vi "Get settings chain.vi"(8 "error in (no error)":errorcluster, 11 "Cascade512Base in":refnum<class "DAQCascade512.lvclass">) -> (0 "error out":errorcluster, 1 "class name":string[](array[string]), 2 "settings":variant[](array[variant]), 3 "Cascade512Base out":refnum<class "DAQCascade512.lvclass">)   [LabVIEW 2012, in "DAQCascade512.lvclass"]
doc: "Returns an array of variants containing the settings clusters of each class in the inheritance chain (lowest child class first), together with an array of all class names in the inheritance chain.\n\nFor classes without settings cluster, the settings chain contains empty variants."
uses:
  DAQCascade512.lvclass
  <vilib>/Distrio/Murmex/Murmex/Murmex.lvclass
  DAQCascade512.lvclass/DAQCascade512.ctl
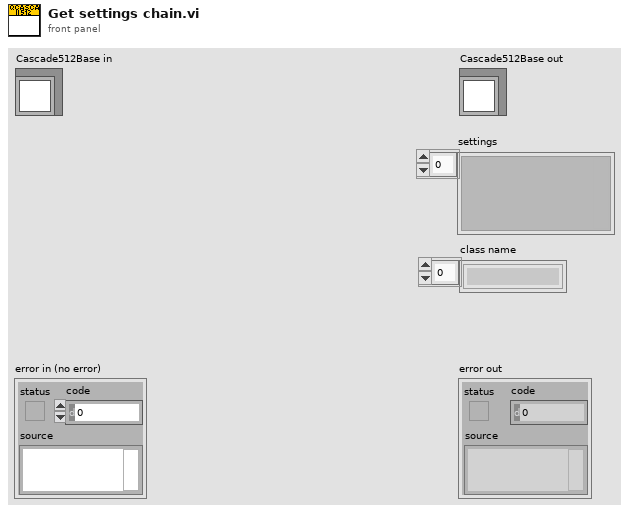
[diagram p1: front panel]
types:
  T1 = typedef "DAQCascade512.lvclass/setting cluster.ctl" = cluster{"number of images":u32, "exposure":dbl}
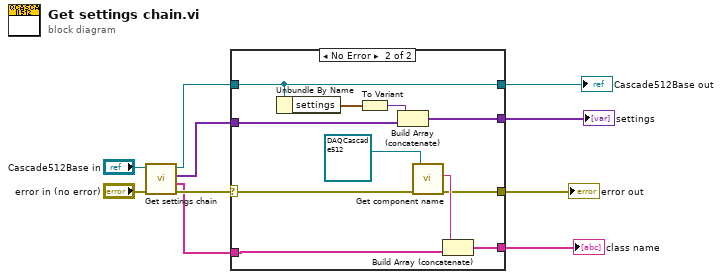
[diagram p0: block diagram]
diagram:
  n1 = call-parent "Get settings chain.vi"("error in (no error)"="error in (no error)", "MurmexBase in"="Cascade512Base in") -> ("error out"=w4:errorcluster, "class name"=w2:string[], "settings"=w6:variant[], "MurmexBase out"=w8:refnum<class "DAQCascade512.lvclass">)  [unwired: 6 in]
  n2 = case shown="No Error" w4 {
    selector: w4 -> [w12 w19]
    tunnel: w8 -> [w14 w17]
    tunnel: [w14 w17] -> w7
    tunnel: w6 -> [w13 w25]
    tunnel: [w13 w24] -> w5
    tunnel: [w12 w18] -> w3
    tunnel: w2 -> [w11 w22]
    tunnel: [w11 w20] -> w1
    frame Error {
    }
    frame No Error {
      n3 = Unbundle By Name(w17) -> ("settings"=w16:T1)
      n4 = To Variant(anything=w16) -> (Variant=w15:variant)
      n5 = Build Array (concatenate)(w15, w25) -> (w24:variant[])
      n6 = call <vilib>:"Get component name.vi"("error in (no error)"=w19, "Murmex in"=refnum<class "DAQCascade512.lvclass"> refnum ("DAQCascade512")) -> ("error out"=w18:errorcluster, "component name"=w21:string)  [unwired: 7 in, 1 out]
      n7 = Build Array (concatenate)(w21, w22) -> (w20:string[])
    }
  }
  "error out" <- w3
  "Cascade512Base out" <- w7
  "settings" <- w5
  "class name" <- w1
